vi "VI Folder Action Template.vi"(8 "error in (no error)":errorcluster, 11 "VI Folder":path) -> (0 "error out":errorcluster, 3 "VI List":path[](array[path]))   [LabVIEW 2016, in "SLL Scripting.lvlib"]
doc: "This template VI to quickly code if any action needs to be done to all VIs in a folder."
uses:
  SLL Scripting.lvlib
  <vilib>/regexp/Match Regular Expression.xnode
panel:
  in  "Exclude Pattern":string
  out "Progress":i32
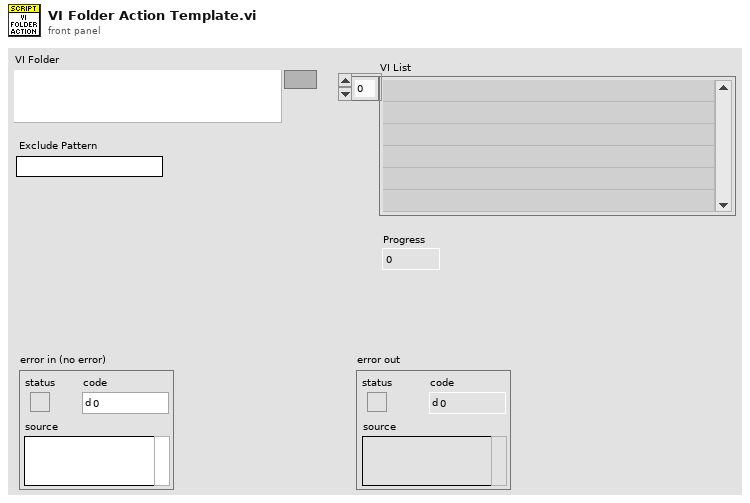
[diagram p1: front panel]
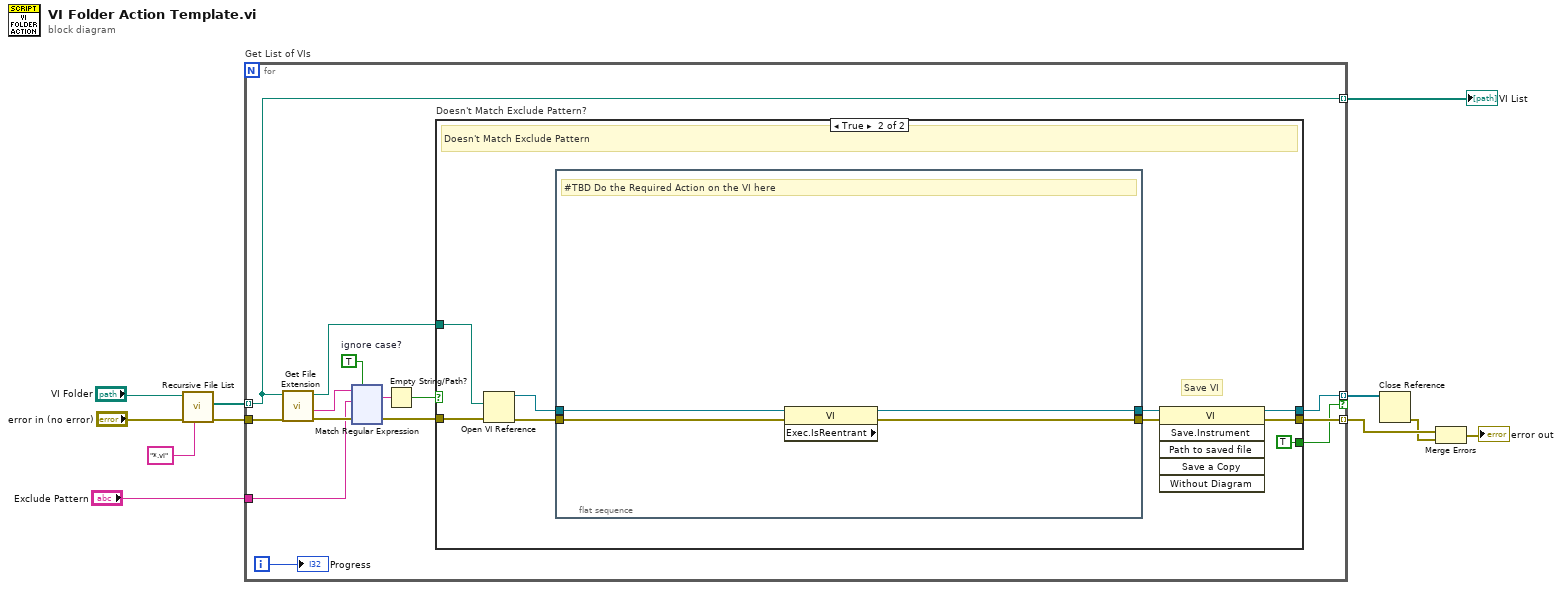
[diagram p0: block diagram]
diagram:
  n1 = call <vilib>:"Recursive File List.vi"("pattern"="*.vi", "error in (no error)"="error in (no error)", "Folder Path"="VI Folder") -> ("error out"=w5:errorcluster, "All Files in Dir"=w8:path[])  [unwired: 4 in, 3 out]
  n2 = for "Get List of VIs" {
    tunnel: [w23] -> w11 mode=indexing if=w14
    tunnel: w8 -> [w12] mode=indexing
    tunnel: [w12] -> w7 mode=indexing
    tunnel: w5 -> [w18]
    tunnel: [w24] -> w4 mode=indexing
    tunnel: "Exclude Pattern" -> [w13]
    i -> [w25]
    w21 = TRUE  # ignore case?
    n3 = call <vilib>:"Get File Extension.vi"("error in (no error)"=w18, "file"=w12) -> ("error out"=w22:errorcluster, "filename without extension"=w20:string, "dup file"=w15:path)  [unwired: 5 in, 2 out]
    n4 = xnode "Match Regular Expression"("input string"=w20, "regular expression"=w13, "error in"=w22, "ignore case? (F)"=w21) -> ("whole match"=w19:string, "error out"=w17:errorcluster)  [unwired: 2 in, 3 out]
    n5 = Empty String/Path?(string/path=w19) -> (empty?=w16:bool)
    n6 = case "Doesn't Match Exclude Pattern?" shown="True" w16 {
      tunnel: [w26 w32] -> w24
      tunnel: [_ w30] -> w23
      tunnel: w17 -> [w26 w29]
      tunnel: w15 -> [_ w28]
      tunnel: [_ TRUE] -> w14
      frame False {
        # "Matches Exclude Pattern, Skip."
      }
      frame True {
        # "Save VI"
        # "Doesn't Match Exclude Pattern"
        n7 = Open VI Reference(vi path=w28, error in (no error)=w29) -> (vi reference=w35:refnum<vi>, error out=w34:errorcluster)  [unwired: 4 in]
        n8 = flat-sequence {
          tunnel: w35 -> [w37]
          tunnel: w34 -> [w39]
          tunnel: [w38] -> w33
          tunnel: [w36] -> w31
          frame #0 {
            # "#TBD Do the Required Action on the VI here"
            n9 = property class="VI" props=["Exec.IsReentrant"](reference=w37, error in=w39) -> (reference out=w36:refnum<vi>, error out=w38:errorcluster)  [unwired: 1 out]
          }
        }
        n10 = invoke class="VI" method="Save.Instrument"(reference=w31, error in=w33) -> (reference out=w30:refnum<vi>, error out=w32:errorcluster)  [unwired: 4 in, 4 out]
      }
    }
    "Progress" <- w25
  }
  "VI List" <- w7
  n11 = Close Reference(reference=w11) -> (error out=w3:errorcluster)  [unwired: 1 in]
  n12 = Merge Errors(w4, w3) -> (→"error out":errorcluster)
